vi "线性公式.vi"(6 "精度":i32=6, 7 "模型":enum32{"线性", "多项式"}(ring), 8 "method":T1 caption="方法" items=["最小二乘", "最小绝对残差", "Bisquare"], 9 "启用":bool[](array[boolean]), 10 "信号值":dbl[](array[numeric]), 11 "标液浓度":dbl[](array[numeric])) -> (0 "Polynomial Coefficients":dbl[](array[numeric]) caption="多项式系数", 1 "XY图":cluster{"X Values":dbl[], "Y Values":dbl[]}[](graph), 2 "r^2":dbl format="%.7g", 3 "拟合方程":string)   [LabVIEW 2016, in "斯坦道原位多参数.lvlib"]
uses:
  <vilib>/Analysis/6fits.llb/Curve Fitting Criteria.ctl
  <vilib>/Analysis/NI_AALPro.lvlib
  <vilib>/gmath/NI_Gmath.lvlib
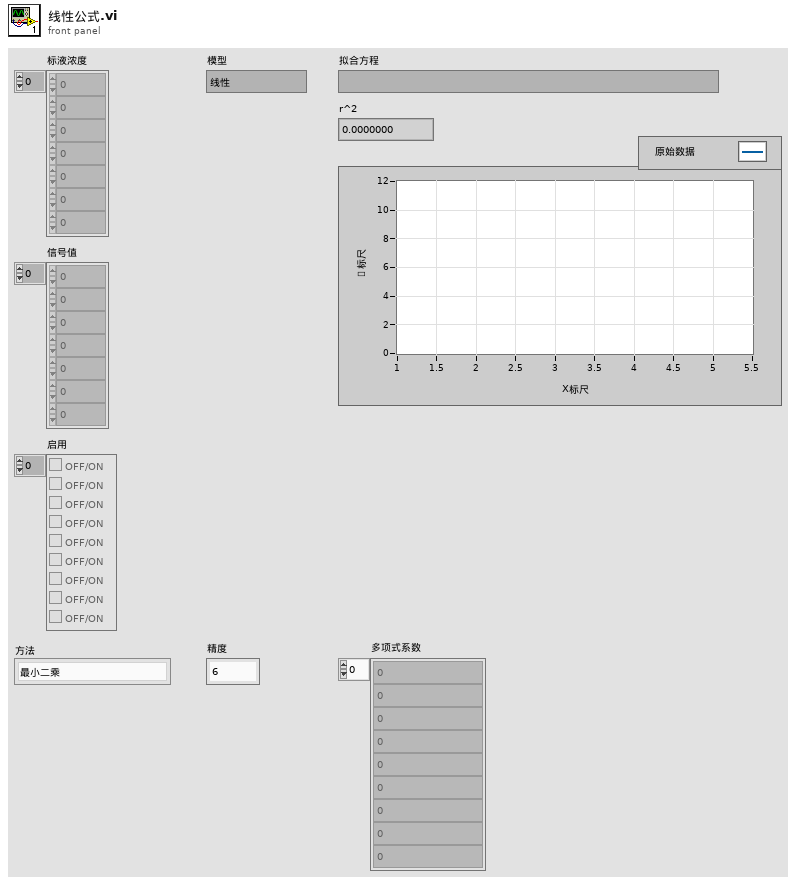
[diagram p1: front panel]
types:
  T1 = typedef "NI_AALPro.lvlib/Curve Fitting Criteria.ctl" = u16
  T2 = enum16{"Linear", "Polynomial", "Exponential", "Power"}
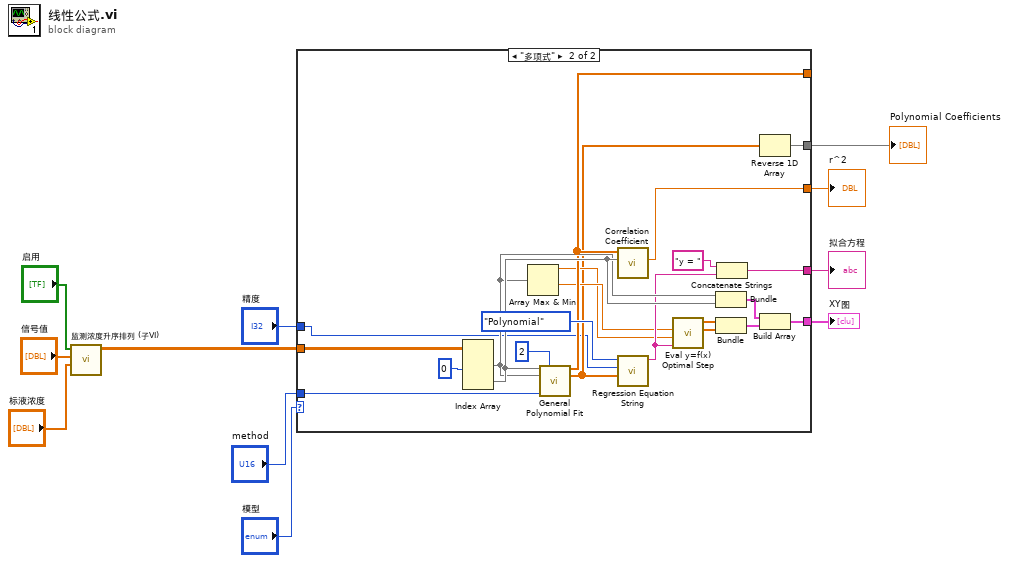
[diagram p0: block diagram]
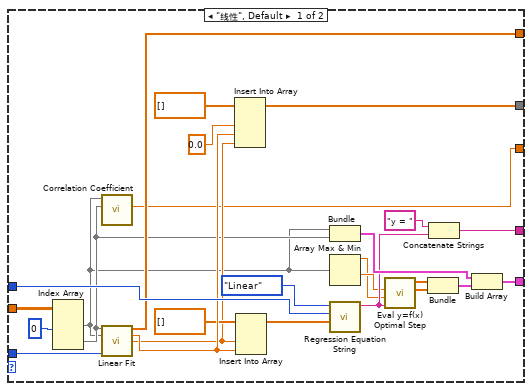
[diagram p2: hidden frame]
diagram:
  n1 = call "监测浓度升序排列 (子VI).vi"("标液浓度"="标液浓度", "滴定数"="信号值", "启用"="启用") -> ("输出数组"=w1:dbl[][])  [unwired: 8 in]
  n2 = case shown="\"多项式\"" "模型" {
    tunnel: w1 -> [w36 w52]
    tunnel: "精度" -> [w29 w38]
    tunnel: [w23 w43] -> _
    tunnel: [w22 w47] -> w6
    tunnel: [w21 w50] -> w5
    tunnel: [w20 w51] -> w4
    tunnel: [w18 w48] -> w3
    tunnel: "method" -> [w15 w44]
    frame "线性", Default {
      n3 = Index Array(array=w36, index (col) #1=0 ("禁用的索引 (列)")) -> (element #1=w16:dbl[], element #2=w17:dbl[])  [unwired: 3 in]
      n4 = call <vilib>:"Correlation Coefficient.vi"("Y"=w17, "X"=w16) -> ("r^2"=w22:dbl)  [unwired: 8 in, 1 out]
      n5 = call <vilib>:"Linear Fit.vi"("Y"=w17, "X"=w16, "method"=w15) -> ("Best Linear Fit"=w23:dbl[], "slope"=w27:dbl, "intercept"=w24:dbl)  [unwired: 8 in, 2 out]
      n6 = Insert Into Array(array=dbl[] [] ("数组"), new element #1=0.0 ("新元素/子数组"), new element #2=w27, new element #3=w24) -> (w18:dbl[])  [unwired: 1 in]
      n7 = Insert Into Array(array=dbl[] [] ("数组"), new element #1=w24, new element #2=w27) -> (w19:dbl[])  [unwired: 1 in]
      n8 = Bundle("输出数组"=w16, "输出数组"=w17) -> (w33:cluster{"输出数组":dbl[], "输出数组":dbl[]})  [unwired: 1 in]
      n9 = Array Max & Min(array=w16) -> (max value=w12:dbl, min value=w13:dbl)  [unwired: 2 out]
      n10 = call "Regression Equation String.vi"("系数"=w19, "精度"=w29, "拟合类型"=T2."Linear") -> ("公式"=w14:string)  [unwired: 8 in]
      n11 = call <vilib>:"Eval y=f(x) Optimal Step.vi"("formula"=w14, "end"=w12, "start"=w13) -> ("Y Values"=w35:dbl[], "X Values"=w34:dbl[])  [unwired: 2 in, 2 out]
      n12 = Bundle("X Values"=w34, "Y Values"=w35) -> (w32:cluster{"X Values":dbl[], "Y Values":dbl[]})  [unwired: 1 in]
      n13 = Concatenate Strings("y = " ("string"), w14) -> (w21:string)
      n14 = Build Array(w33, w32) -> (w20:cluster{"X Values":dbl[], "Y Values":dbl[]}[])
    }
    frame "多项式" {
      n15 = Index Array(array=w52, index (col) #1=0 ("禁用的索引 (列)")) -> (element #1=w45:dbl[], element #2=w46:dbl[])  [unwired: 3 in]
      n16 = Array Max & Min(array=w45) -> (max value=w40:dbl, min value=w41:dbl)  [unwired: 2 out]
      n17 = call <vilib>:"General Polynomial Fit.vi"("Y"=w46, "polynomial order"=2, "X"=w45, "method"=w44) -> ("Best Polynomial Fit"=w43:dbl[], "Polynomial Coefficients"=w39:dbl[])  [unwired: 8 in, 2 out]
      n18 = call <vilib>:"Correlation Coefficient.vi"("Y"=w46, "X"=w43) -> ("r^2"=w47:dbl)  [unwired: 8 in, 1 out]
      n19 = call "Regression Equation String.vi"("系数"=w39, "精度"=w38, "拟合类型"=T2."Polynomial") -> ("公式"=w42:string)  [unwired: 8 in]
      n20 = call <vilib>:"Eval y=f(x) Optimal Step.vi"("formula"=w42, "end"=w40, "start"=w41) -> ("Y Values"=w58:dbl[], "X Values"=w57:dbl[])  [unwired: 2 in, 2 out]
      n21 = Bundle("输出数组"=w45, "输出数组"=w46) -> (w56:cluster{"输出数组":dbl[], "输出数组":dbl[]})  [unwired: 1 in]
      n22 = Bundle("X Values"=w57, "Y Values"=w58) -> (w55:cluster{"X Values":dbl[], "Y Values":dbl[]})  [unwired: 1 in]
      n23 = Concatenate Strings("y = " ("string"), w42) -> (w50:string)
      n24 = Reverse 1D Array(array=w39) -> (reversed array=w48:dbl[])
      n25 = Build Array(w56, w55) -> (w51:cluster{"X Values":dbl[], "Y Values":dbl[]}[])
    }
  }
  "r^2" <- w6
  "拟合方程" <- w5
  "XY图" <- w4
  "Polynomial Coefficients" <- w3
